vi "CSDB_SVEdit.get substring indexes.vi"(1 "stringArray":string[](array[string]), 4 "subString":string) -> (15 "indexes":i32[](array[numeric]))   [LabVIEW 2014, in "CSDB_SVEdit.lvlib"]
doc: "Checks array elements for a substring and returns all array indexes, where the substring has been found."
uses:
  CSDB_SVEdit.lvlib
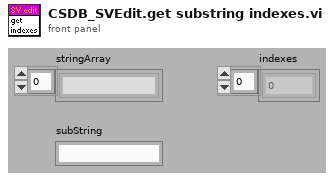
[diagram p1: front panel]
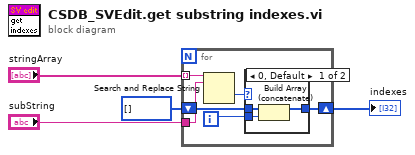
[diagram p0: block diagram]
diagram:
  n1 = for {
    tunnel: "stringArray" -> [w6] mode=indexing
    tunnel: "subString" -> [w7]
    shift-right: [w9] -> w1
    shift-left: i32[] [] -> [w10]
    i -> [w8]
    n2 = Search and Replace String(input string=w6, search string=w7) -> (offset past replacement=w5:i32)  [unwired: 6 in, 3 out]
    n3 = case shown="0, Default" w5 {
      tunnel: w10 -> [w13 w14]
      tunnel: [w12 w14] -> w9
      tunnel: w8 -> [w11 _]
      frame 0, Default {
        n4 = Build Array (concatenate)(w13, w11) -> (w12:i32[])
      }
      frame -1 {
      }
    }
  }
  "indexes" <- w1
